vi "add_point32.vi"(6 "Point32":cluster{"x":dbl, "y":dbl, "z":dbl}, 7 "msg in":string) -> (3 "msg out":string)   [LabVIEW 2012]
doc: "Flattens a point 32 into a message"
uses:
  <userlib>/ROS for LabVIEW Software/ROS/MessageBuilding/std_msgs/subs/float32Scalar.vi
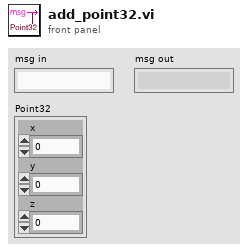
[diagram p1: front panel]
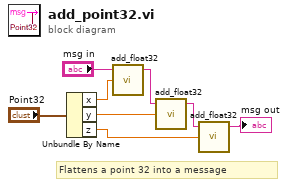
[diagram p0: block diagram]
diagram:
  # "Flattens a point 32 into a message"
  n1 = Unbundle By Name("Point32") -> ("x"=w7:dbl, "y"=w4:dbl, "z"=w2:dbl)
  n2 = call-poly <userlib>:"add_float32.vi"("Numeric"=w7, "msg in"="msg in") -> ("msg out"=w5:string)  [unwired: 3 in]
  n3 = call-poly <userlib>:"add_float32.vi"("Numeric"=w4, "msg in"=w5) -> ("msg out"=w3:string)  [unwired: 3 in]
  n4 = call-poly <userlib>:"add_float32.vi"("Numeric"=w2, "msg in"=w3) -> ("msg out"=→"msg out":string)  [unwired: 3 in]
